vi "showError.vi"(3 "message":string, 5 "Error IN":errorcluster) -> (2 "Error OUT":errorcluster)   [LabVIEW 2010]
uses:
  <vilib>/Utility/error.llb/DialogType.ctl
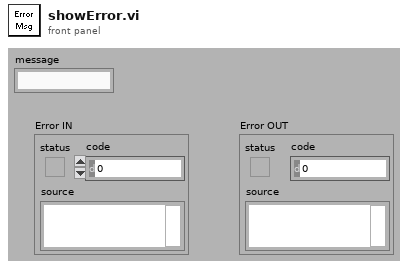
[diagram p1: front panel]
types:
  T1 = typedef "DialogType.ctl" = u16
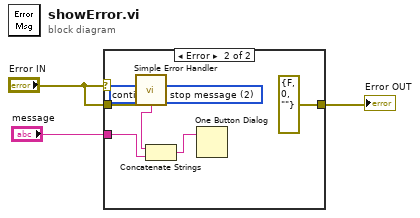
[diagram p0: block diagram]
diagram:
  n1 = case shown="Error" "Error IN" {
    tunnel: [w4 errorcluster {"status"=FALSE, "code"=0, "source"=""} ("Error OUT")] -> w3
    tunnel: "Error IN" -> [w4 w9]
    tunnel: "message" -> [_ w6]
    frame No Error {
    }
    frame Error {
      w5 = T1 2 items=["no dialog", "OK message", "continue or stop message", "OK message + warnings", "continue/stop + warnings"] ("type of dialog (OK msg:1)")
      n2 = call <vilib>:"Simple Error Handler.vi"("type of dialog (OK msg:1)"=w5, "error in (no error)"=w9) -> ("message"=w7:string)  [unwired: 3 in, 4 out]
      n3 = Concatenate Strings(w7, w6) -> (w8:string)
      n4 = One Button Dialog(message=w8) -> ()  [unwired: 1 in, 1 out]
    }
  }
  "Error OUT" <- w3
